vi "Simple Read.vi"(4 "Class":refnum<class "Abs_U32 Integer.lvclass">) -> (1 "Value":u32)   [LabVIEW 2021, in "Abs_U32 Integer.lvclass"]
uses:
  Abs_U32 Integer.lvclass
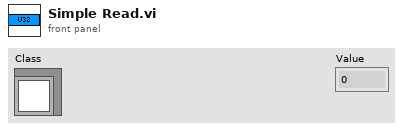
[diagram p1: front panel]
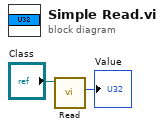
[diagram p0: block diagram]
diagram:
  n1 = call-dynamic "Read.vi"("Double Float.lvclass_340760 in"="Class") -> ("Value"=→"Value":u32)  [unwired: 8 in, 2 out]
